vi "Nested Aliases.vi"(11 "Dev Actor in":refnum<class "Dev Actor.lvclass">) -> (2 "Nested Aliases":string[](array[string]))   [LabVIEW 2021, in "Dev Actor.lvlib" / "Dev Actor.lvclass"]
uses:
  Dev Actor.lvclass
  Dev Actor.lvclass/Dev Actor.ctl
  Actor/Queue Actor/Queue Actor.lvclass
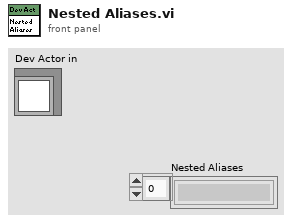
[diagram p1: front panel]
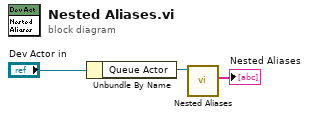
[diagram p0: block diagram]
diagram:
  n1 = Unbundle By Name("Dev Actor in") -> ("Queue Actor"=w2:refnum<class "Queue Actor.lvclass">)
  n2 = call-dynamic "Nested Aliases.vi"("Queue Actor in"=w2) -> ("Nested Aliases"=→"Nested Aliases":string[])  [unwired: 10 in]
